vi "Write IP_Address.vi"(8 "error in (no error)":errorcluster, 10 "IP_Address":string, 11 "MonSys_Client_Actor in":refnum<class "MonSys_Client_Actor.lvclass">) -> (0 "error out":errorcluster, 3 "MonSys_Client_Actor out":refnum<class "MonSys_Client_Actor.lvclass">)   [LabVIEW 2018, in "MonSys_Client_Actor.lvlib" / "MonSys_Client_Actor.lvclass"]
uses:
  MonSys_Client_Actor.lvclass
  MonSys_Client_Actor.lvclass/MonSys_Client_Actor.ctl
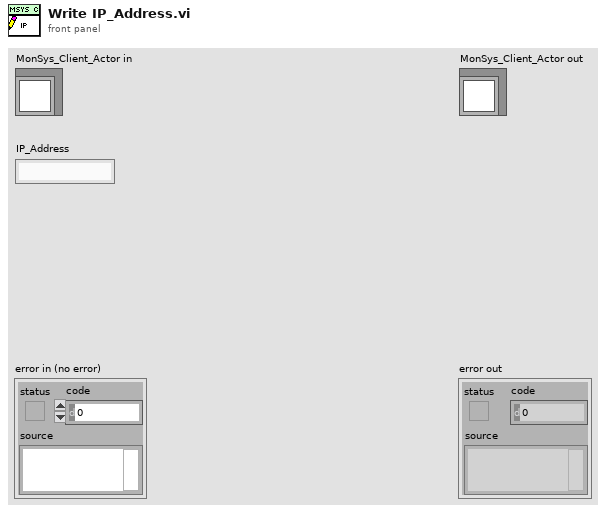
[diagram p1: front panel]
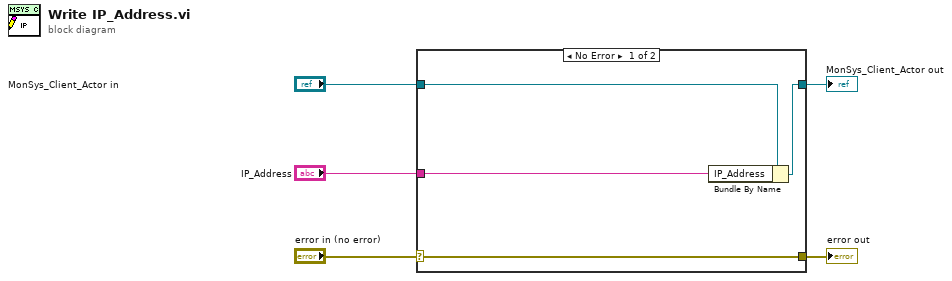
[diagram p0: block diagram]
diagram:
  n1 = case shown="No Error" "error in (no error)" {
    selector: "error in (no error)" -> [w9 w10]
    tunnel: [w9 w10] -> w4
    tunnel: [w7 w11] -> w2
    tunnel: "MonSys_Client_Actor in" -> [w8 w11]
    tunnel: "IP_Address" -> [w6 _]
    frame No Error {
      n2 = Bundle By Name(cluster=w8, "IP_Address"=w6) -> (w7:refnum<class "MonSys_Client_Actor.lvclass">)
    }
    frame Error {
    }
  }
  "error out" <- w4
  "MonSys_Client_Actor out" <- w2
